vi "JSON to LVObject.vi"(7 "JSON Serializable Serializer in":refnum<class "JSON Serializable Serializer.lvclass">, 8 "error in (no error)":errorcluster, 9 "Object Type":refnum<class>, 10 "Offset":i32, 11 "JSON":string) -> (0 "error out":errorcluster, 1 "Object":refnum<class>)   [LabVIEW 2017, in "JSON Serializable Serializer.lvclass"]
uses:
  JSON Serializable Serializer.lvclass
  C:/Program Files (x86)/National Instruments/LabVIEW 2017/vi.lib/JDP Science/JSONtext/LVClass Serializer/JSONtext LVClass Serializer.lvclass
  JSON Serializable/JSON Serializable.lvclass
  Default Serialization Binder/Default Serialization Binder.lvclass
  <vilib>/JDP Science/JSONtext/Delete.vi
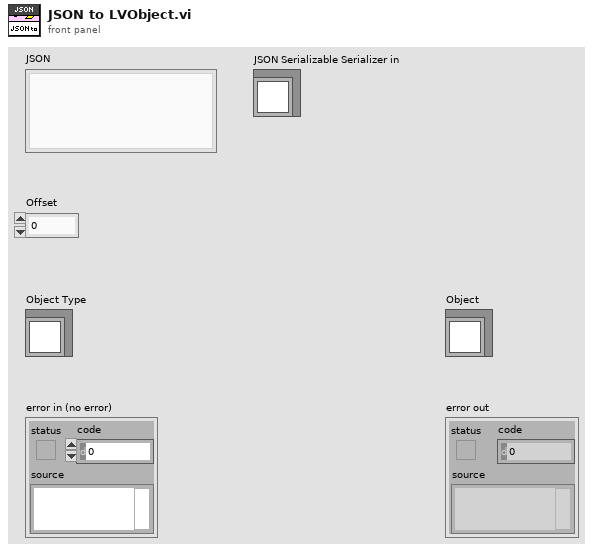
[diagram p1: front panel]
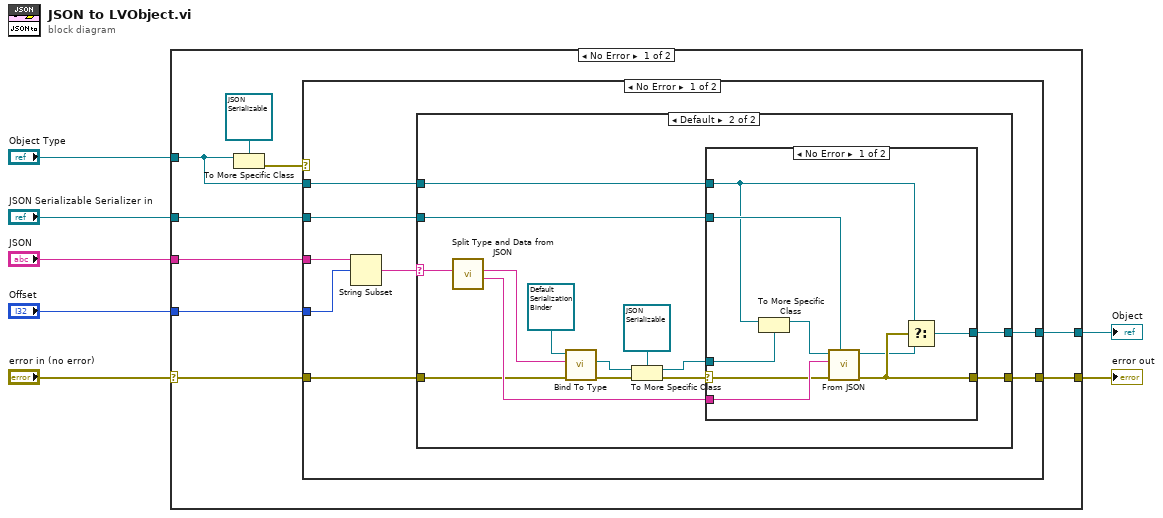
[diagram p0: block diagram]
diagram:
  n1 = case shown="No Error" "error in (no error)" {
    selector: "error in (no error)" -> [w10 w55]
    tunnel: "JSON Serializable Serializer in" -> [w16 _]
    tunnel: [w15 w54] -> w6
    tunnel: "JSON" -> [w14 _]
    tunnel: [w9 w55] -> w3
    tunnel: "Object Type" -> [w11 w54]
    tunnel: "Offset" -> [w8 _]
    frame No Error {
      n2 = To More Specific Class(target class=refnum<class "JSON Serializable.lvclass"> refnum ("JSON Serializable.lvclass"), reference=w11) -> (error out=w12:errorcluster)  [unwired: 1 in, 1 out]
      n3 = case shown="No Error" w12 {
        tunnel: w16 -> [w24 _]
        tunnel: [w23 w53] -> w15
        tunnel: w14 -> [w19 _]
        tunnel: w11 -> [w20 w53]
        tunnel: w10 -> [w22 w52]
        tunnel: [w21 w52] -> w9
        tunnel: w8 -> [w18 _]
        frame No Error {
          n4 = String Subset(string=w19, offset (0)=w18) -> (substring=w17:string)  [unwired: 1 in]
          n5 = case shown="Default" w17 {
            selector: w17 -> [_ w36]
            tunnel: w24 -> [_ w40]
            tunnel: [w25 w29] -> w23
            tunnel: w22 -> [w26 w32]
            tunnel: [w26 w30] -> w21
            tunnel: w20 -> [w25 w28]
            frame "" {
            }
            frame Default {
              n6 = call "Split Type and Data from JSON.vi"("<JSON>"=w36) -> ("Data"=w39:string, "Type"=w37:string)  [unwired: 9 in]
              n7 = call-dynamic "Bind To Type.vi"("error in (no error)"=w32, "Type Name"=w37, "Default Serialization Binder in"=refnum<class "Default Serialization Binder.lvclass"> refnum ("Default Serialization Binder")) -> ("error out"=w31:errorcluster, "Type"=w35:refnum<class>)  [unwired: 6 in, 1 out]
              n8 = To More Specific Class(target class=refnum<class "JSON Serializable.lvclass"> refnum ("JSON Serializable.lvclass"), reference=w35, error in=w31) -> (specific class reference=w34:refnum<class "JSON Serializable.lvclass">, error out=w27:errorcluster)
              n9 = case shown="No Error" w27 {
                selector: w27 -> [w42 w50]
                tunnel: w40 -> [w49 _]
                tunnel: w39 -> [w48 _]
                tunnel: w34 -> [w46 _]
                tunnel: [w45 w50] -> w30
                tunnel: [w44 w51] -> w29
                tunnel: w28 -> [w43 w51]
                frame No Error {
                  n10 = To More Specific Class(target class=w46, reference=w43) -> (specific class reference=w47:refnum<class "JSON Serializable.lvclass">)  [unwired: 1 in, 1 out]
                  n11 = call-dynamic "From JSON.vi"("LVClass Serializer"=w49, "error in (no error)"=w42, "<JSON>"=w48, "JSON Serializable in"=w47) -> ("error out"=w45:errorcluster, "JSON Serializable out"=w41:refnum<class "JSON Serializable.lvclass">)  [unwired: 6 in]
                  n12 = Select(t=w43, s=w45, f=w41) -> (s? t:f=w44:refnum<class>)
                }
                frame Error {
                }
              }
            }
          }
        }
        frame Error {
        }
      }
    }
    frame Error {
    }
  }
  "error out" <- w3
  "Object" <- w6
